vi "Sec2MinSec.vi"(11 "duration (s)":string) -> (3 "duration (mm:ss)":string)   [LabVIEW 2015]
panel:
  out "value":dbl
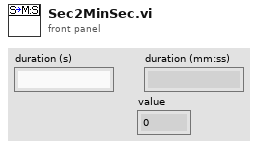
[diagram p1: front panel]
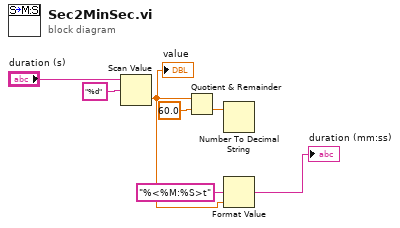
[diagram p0: block diagram]
diagram:
  n1 = Scan Value(string="duration (s)", format string="%d") -> (value=w3:dbl)  [unwired: 1 in, 1 out]
  "value" <- w3
  n2 = Quotient & Remainder(x=w3, y=60.0) -> (floor(x/y)=w5:dbl)  [unwired: 1 out]
  n3 = Number To Decimal String(number=w5) -> ()  [unwired: 1 in, 1 out]
  n4 = Format Value(format string="%<%M:%S>t", value (0)=w3) -> (output string=→"duration (mm:ss)":string)  [unwired: 1 in]
